vi "OE1022D_Configure Harmonic.vi"(0 "VISA resource name":refnum<visa-resource-name>, 1 "OE1022D A/B":u8(ring) items=["Channel A", "Channel B"], 2 "Harmonic 1":u16=1, 3 "Harmonic 2":u16=1, 5 "error in (no error)":errorcluster) -> (14 "VISA resource name out":refnum<visa-resource-name>, 19 "error out":errorcluster)   [LabVIEW 2022 SP3]
doc: "Configures the reference source and the internal oscillator."
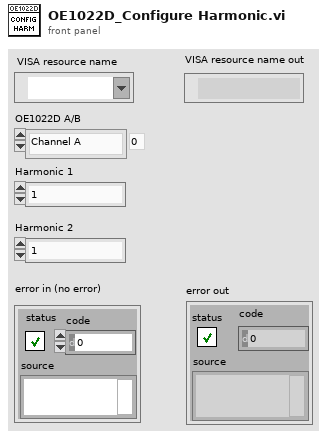
[diagram p1: front panel]
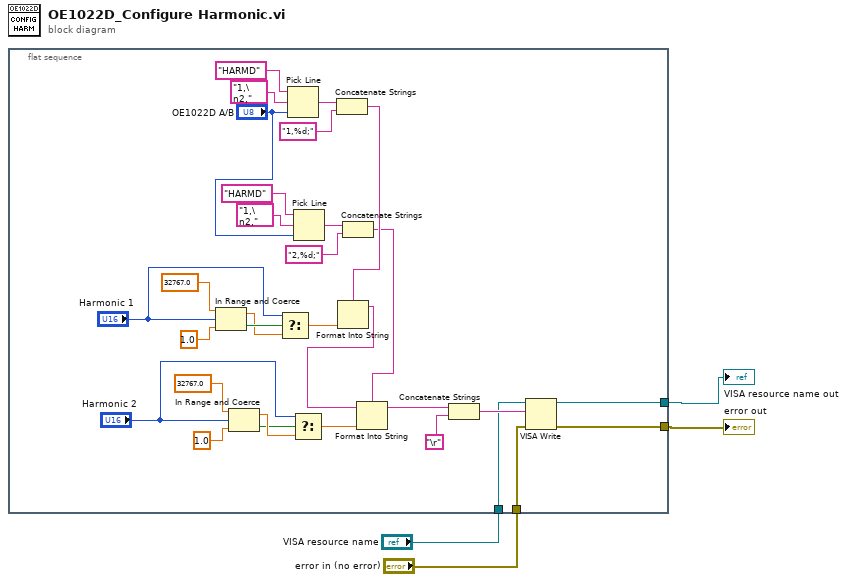
[diagram p0: block diagram]
diagram:
  n1 = flat-sequence {
    tunnel: "error in (no error)" -> [w32]
    tunnel: "VISA resource name" -> [w33]
    tunnel: [w17] -> w4
    tunnel: [w16] -> w3
    frame #0 {
      n2 = In Range and Coerce(upper limit=32767.0 ("t"), x="Harmonic 1", lower limit=1.0 ("t")) -> (coerced(x)=w26:dbl, In Range?=w27:bool)
      n3 = In Range and Coerce(upper limit=32767.0 ("t"), x="Harmonic 2", lower limit=1.0 ("t")) -> (coerced(x)=w25:dbl, In Range?=w24:bool)
      n4 = Select(t="Harmonic 1", s=w27, f=w26) -> (s? t:f=w31:dbl)
      n5 = Pick Line(string ("")="HARMD", multi-line string="1,\n2,", line index="OE1022D A/B") -> (output string=w9:string)
      n6 = Select(t="Harmonic 2", s=w24, f=w25) -> (s? t:f=w21:dbl)
      n7 = Pick Line(string ("")="HARMD", multi-line string="1,\n2,", line index="OE1022D A/B") -> (output string=w12:string)
      n8 = Concatenate Strings(w9, "1,%d;" ("字符串")) -> (w6:string)
      n9 = Format Into String(format string=w6, w31) -> (resulting string=w19:string)  [unwired: 2 in, 1 out]
      n10 = Concatenate Strings(w12, "2,%d;" ("字符串")) -> (w5:string)
      n11 = Format Into String(format string=w5, initial string=w19, w21) -> (resulting string=w18:string)  [unwired: 1 in, 1 out]
      n12 = Concatenate Strings(w18, "\r") -> (w34:string)
      n13 = VISA Write(VISA resource name=w33, write buffer=w34, error in (no error)=w32) -> (VISA resource name out=w17:refnum<visa-resource-name>, error out=w16:errorcluster)  [unwired: 1 out]
    }
  }
  "error out" <- w3
  "VISA resource name out" <- w4
